vi "main.vi"() -> ()   [LabVIEW 2018]
uses:
  <vilib>/daq.io/MQTT LabVIEW Client/Controls/QoS.ctl
  <vilib>/daq.io/MQTT LabVIEW Client/MQTT_Functions.lvlib
panel:
  in  "QoS":T1
  in  "portNo":i32
  in  "txtClientID":string
  out "error out":errorcluster
  in  "error in (no error)":errorcluster
  in  "txtMessage":string
  in  "txtTopicToPublish":string
  out "boolPublished":bool
  in  "btnPublish":bool
  in  "txtTopicToSubscribe":string
  out "boolSubscribed":bool
  in  "btnSubscribe":bool
  in  "btnDisconnect":bool
  in  "txtIP":string
  in  "btnConnect":bool
  out "boolConnection":bool
  in  "stop":bool
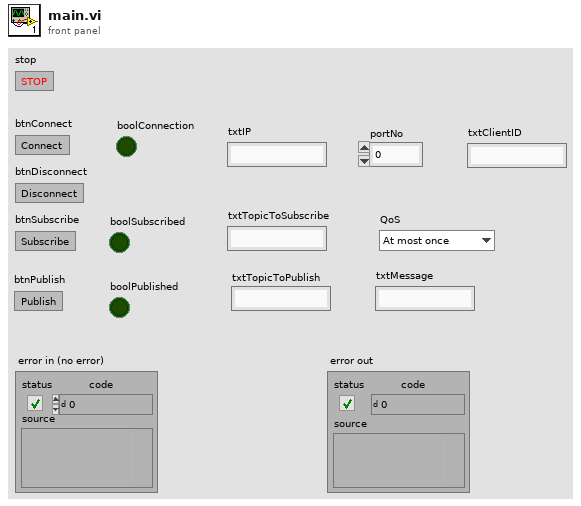
[diagram p1: front panel]
types:
  T1 = typedef "MQTT_Functions.lvlib/QoS.ctl" = enum8{"At most once", "At least once", "Exactly once", "Reserved"}
  T2 = typedef "MQTT_Functions.lvlib/Connection_Return_Codes.ctl" = enum16{"Connection accepted", "Connection refused: unacceptable protocol version", "Connection refused: identifier rejected", "Connection refused: Server unavailable", "Connection refused: bad user name or password", "Connection refused: not authorized"}
  T3 = cluster{"txtTopicToSubscribe":string, "QoS":T1}[]
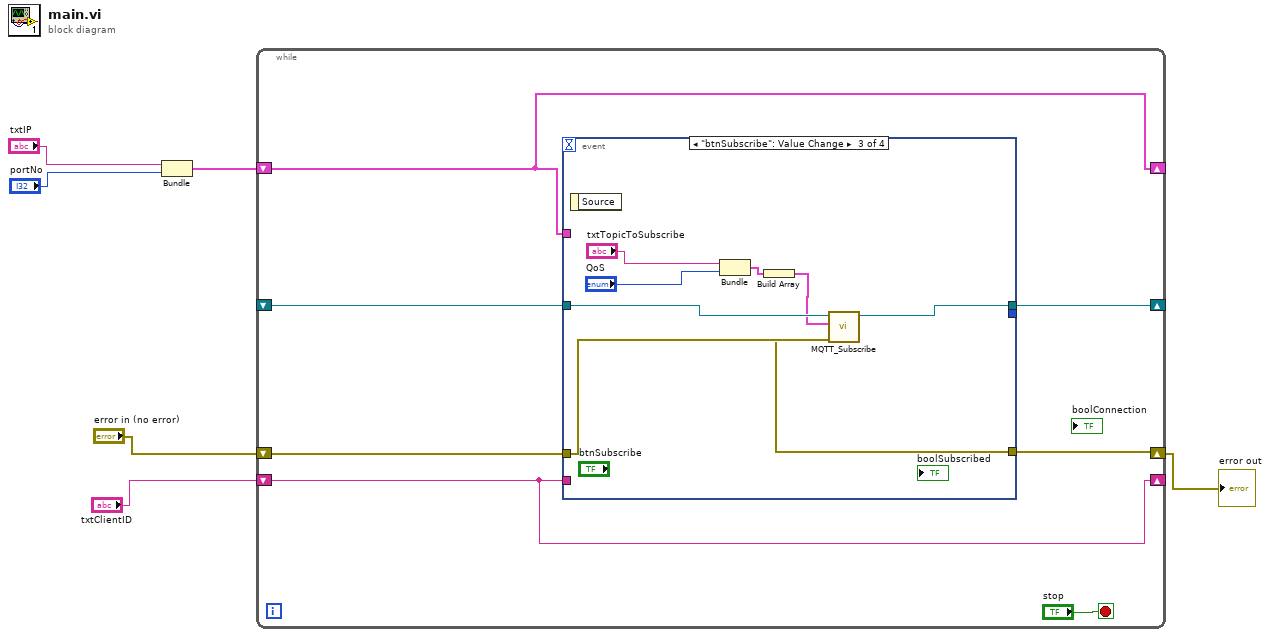
[diagram p0: block diagram]
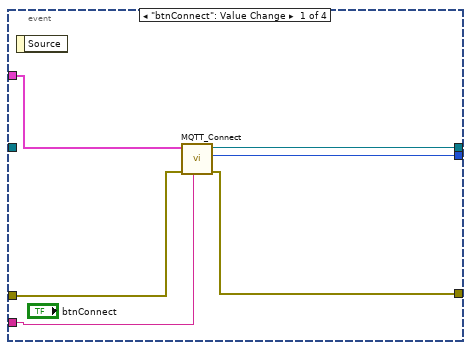
[diagram p2: hidden frame]
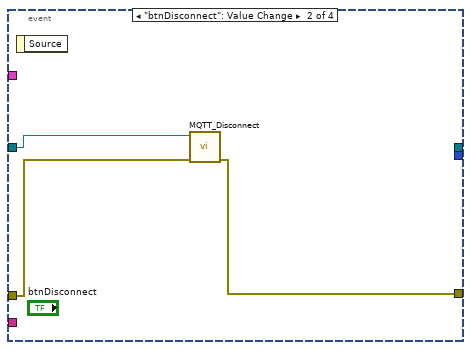
[diagram p3: hidden frame]
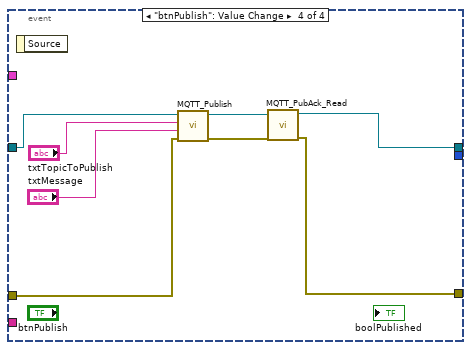
[diagram p4: hidden frame]
diagram:
  n1 = Bundle("txtIP"="txtIP", "portNo"="portNo") -> (w4:cluster{"txtIP":string, "portNo":i32})  [unwired: 1 in]
  n2 = while {
    shift-right: [w11] -> _
    shift-left: _ -> [w12]
    shift-right: [w10] -> _
    shift-left: w4 -> [w10]
    shift-right: [w8] -> w1
    shift-left: "error in (no error)" -> [w9]
    shift-right: [w7] -> _
    shift-left: "txtClientID" -> [w7]
    stop <- "stop" stop-if-true
    n3 = event shown="[2] \"btnSubscribe\": Value Change" {
      selector: _ -> [_ _ _ _]
      dyn-events: _ -> [_ _ _ _]
      timeout: _ -> [_ _ _ _]
      tunnel: [w19 w20 w28 w34] -> w8
      tunnel: w9 -> [w18 w21 w29 w37]
      tunnel: [w17 _ _ _] -> _
      tunnel: [w16 _ w27 w33] -> w11
      tunnel: w12 -> [_ w22 w30 w38]
      tunnel: w7 -> [w15 _ _ _]
      tunnel: w10 -> [w14 _ _ _]
      event "btnConnect": Value Change {
        n4 = event-data() -> ()  [unwired: 1 in, 1 out]
        n5 = call <vilib>:"MQTT_Connect.vi"("Client ID"=w15, "error in (no error)"=w18, "MQTT Broker"=w14) -> ("error out"=w19:errorcluster, "Connection Status"=w17:T2, "connection ID out"=w16:refnum<k5>)  [unwired: 6 in]
      }
      event "btnDisconnect": Value Change {
        n6 = event-data() -> ()  [unwired: 1 in, 1 out]
        n7 = call <vilib>:"MQTT_Disconnect.vi"("error in (no error)"=w21, "connection ID"=w22) -> ("error out"=w20:errorcluster)  [unwired: 9 in]
      }
      event "btnSubscribe": Value Change {
        n8 = event-data() -> ()  [unwired: 1 in, 1 out]
        n9 = Bundle("txtTopicToSubscribe"="txtTopicToSubscribe", "QoS"="QoS") -> (w26:cluster{"txtTopicToSubscribe":string, "QoS":T1})  [unwired: 1 in]
        n10 = Build Array(w26) -> (w23:T3)
        n11 = call <vilib>:"MQTT_Subscribe.vi"("error in (no error)"=w29, "Subscription Info Array"=w23, "connection ID"=w30) -> ("error out"=w28:errorcluster, "connection ID out"=w27:refnum<k5>)  [unwired: 7 in]
      }
      event "btnPublish": Value Change {
        n12 = event-data() -> ()  [unwired: 1 in, 1 out]
        n13 = call <vilib>:"MQTT_Publish.vi"("error in (no error)"=w37, "Message to be published"="txtMessage", "Topic"="txtTopicToPublish", "connection ID"=w38) -> ("error out"=w35:errorcluster, "connection ID out"=w36:refnum<k5>)  [unwired: 6 in]
        n14 = call <vilib>:"MQTT_PubAck_Read.vi"("error in (no error)"=w35, "connection ID"=w36) -> ("error out"=w34:errorcluster, "connection ID out"=w33:refnum<k5>)  [unwired: 7 in, 1 out]
      }
    }
  }
  "error out" <- w1
